vi "delta&2400 measure.vi"(0 "6221":refnum<visa-resource-name>, 5 "2400":refnum<visa-resource-name>, 9 "Timeout":u32, 11 "错误输出":errorcluster) -> (3 "source current":string, 4 "6221":refnum<visa-resource-name>, 6 "2400 resource name out":refnum<visa-resource-name>, 8 "2400":string[](array[string]), 10 "6221":string, 14 "compliance?":bool, 15 "error out":errorcluster)   [LabVIEW 2019, in "nematic.lvlib"]
uses:
  SubVI/nematic.lvlib
  lib/Keithley 622x/Configure/Format/Typedefs/KE622x -- Optional Meas Elements.ctl
  lib/Keithley 622x/Keithley 622x.lvlib
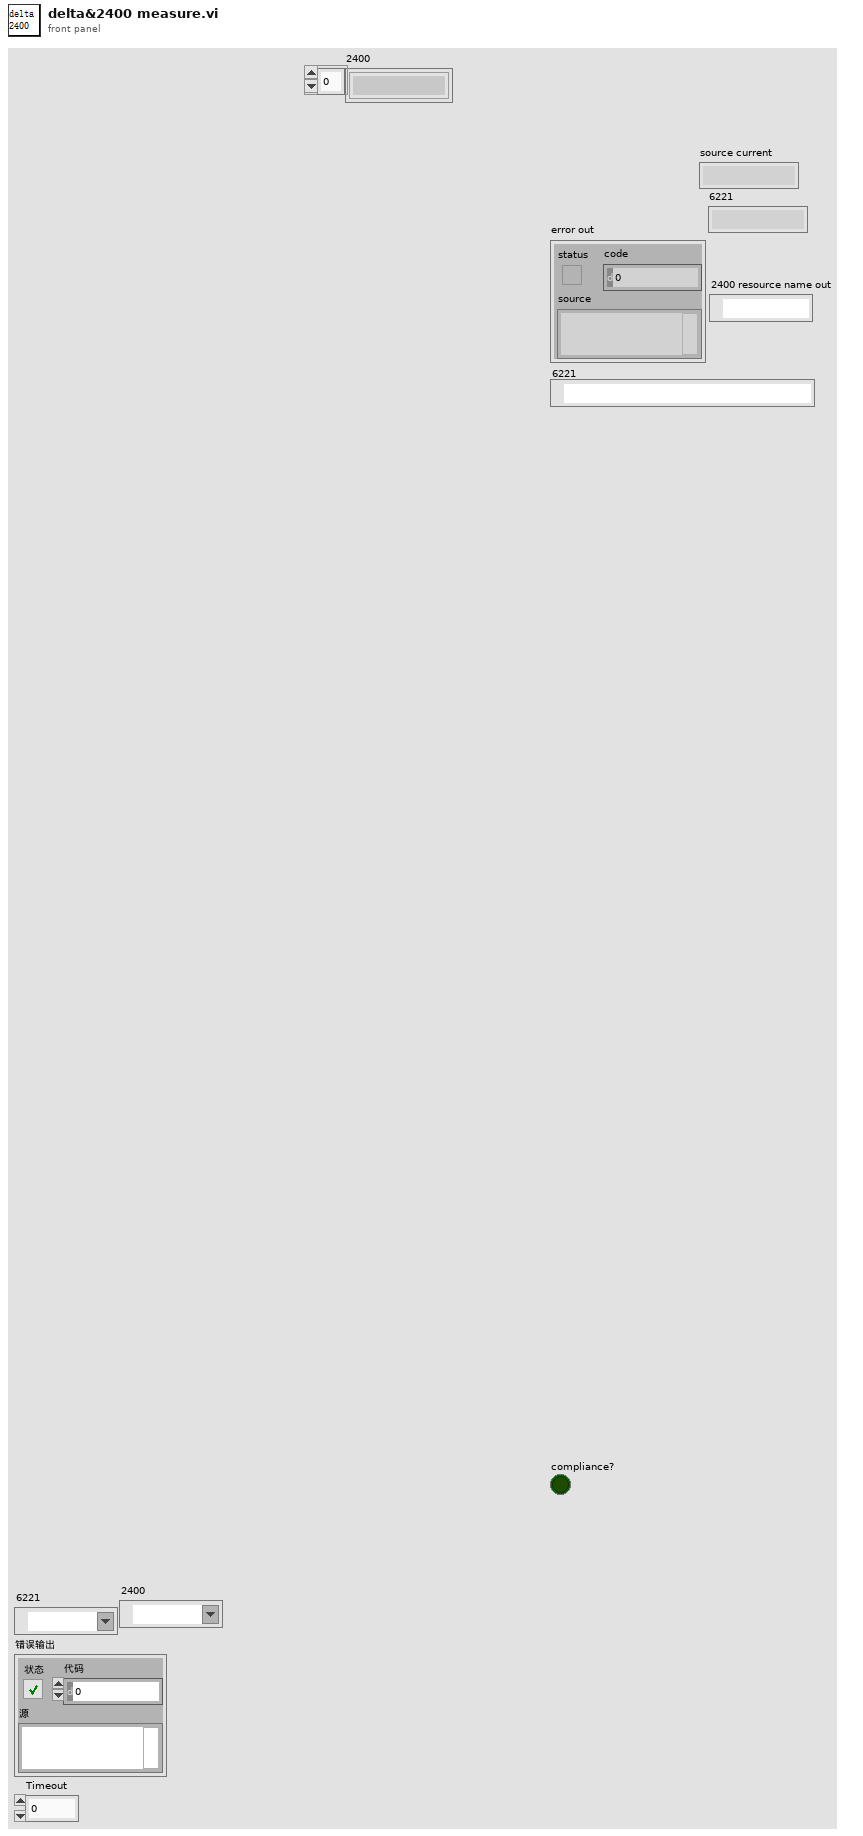
[diagram p1: front panel]
types:
  T1 = typedef "Keithley 622x.lvlib/KE622x -- Optional Meas Elements.ctl" = cluster{"Timstamp?":bool, "Reading Num?":bool, "Source Value?":bool, "Compliance?":bool, "Average Voltage?":bool}
  T2 = typedef "Keithley 622x.lvlib/KE622x -- Meas Event Reg State.ctl" = cluster{"B0, ROF:  KE2182A Delta Reading Overflow Event?":bool, "B1, Int:  Interlock OK Event?":bool, "B2, Temp:  Over Temperature Event?":bool, "B3, Comp:  Compliance Event?":bool, "B5, RAV:  Delta Reading Available Event?":bool, "B6, TN:  User Defined Reading Number Stored In Buffer Event?":bool, "B7, BAV:  At Least 2 Readings Stored In Buffer Event?":bool, "B12, BQF:  Buffer Quarter Full Event?":bool, "B8, BHF:  Buffer Half Full Event?":bool, "B13, B3QF:  Buffer 3/4 Full Event?":bool, "B9, BFL:  Buffer Full Event?":bool}
  T3 = typedef "Keithley 622x.lvlib/KE622x -- Trace Buf.ctl" = cluster{"Additional Valid Arrays":T1, "Reading Num":u32[], "Timestamp (secs)":sgl[], "Source Val (A)":sgl[], "Reading":sgl[], "Average Voltage (V)":sgl[], "Compliance?":bool[]}
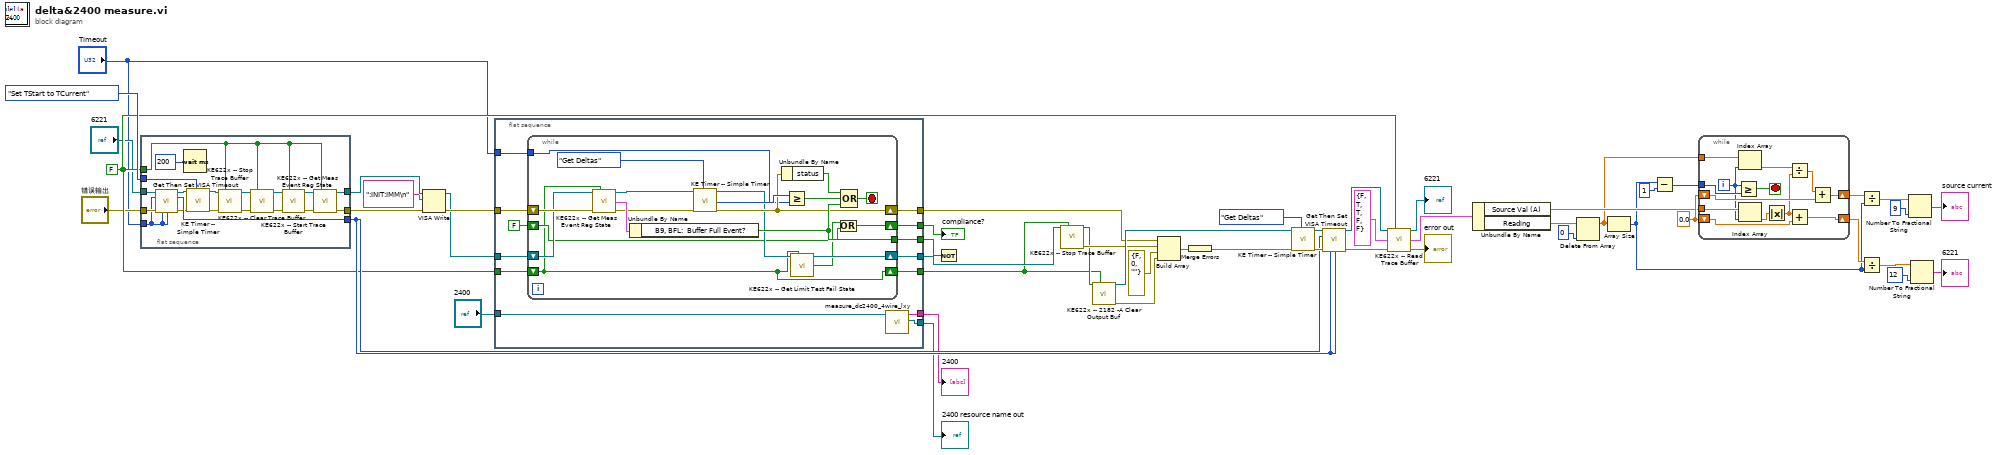
[diagram p0: block diagram]
diagram:
  w20 = FALSE ("Check For SCPI Errors? (T) 2")
  w33 = sgl 0.0 ("Numeric")
  n1 = flat-sequence {
    tunnel: enum16{"Set TStart to TCurrent", "Get Deltas"}."Set TStart to TCurrent" ("Action") -> [w66]
    tunnel: [w53] -> w44
    tunnel: [w52] -> w43
    tunnel: [w61] -> w36
    tunnel: "6221" -> [w58]
    tunnel: w20 -> [w57]
    tunnel: "错误输出" -> [w56]
    tunnel: "Timeout" -> [w55]
    frame #0 {
      n2 = call "Get Then Set VISA Timeout.vi"("VISA Resource Name In"=w58, "New Timeout (msecs)"=w55, "error in (no error)"=w56, "Max Timeout (300 secs)"=w55, "Min Timeout (3 secs)"=w55) -> ("VISA Resource Name Out (dupl)"=w60:refnum<visa-resource-name>, "Old Timeout (msecs)"=w61:u32, "error out"=w59:errorcluster)  [unwired: 7 in, 1 out]
      n3 = Wait (ms)(milliseconds to wait=u32 200) -> ()  [unwired: 1 out]
      n4 = call "KE Timer -- Simple Timer.vi"("Resource In"=w60, "error in (no error)"=w59, "Action"=w66) -> ("Resource Out (dupl)"=w65:refnum<visa-resource-name>, "error out (dupl)"=w64:errorcluster)  [unwired: 7 in, 8 out]
      n5 = call "KE622x -- Stop Trace Buffer.vi"("Resource In"=w65, "Check For SCPI Errors? (T)"=w57, "error in (no error)"=w64) -> ("Resource Out (dupl)"=w70:refnum<visa-resource-name>, "error out"=w69:errorcluster)  [unwired: 11 in]
      n6 = call "KE622x -- Clear Trace Buffer.vi"("Resource In"=w70, "Check For SCPI Errors? (T)"=w57, "error in (no error)"=w69) -> ("Resource Out (dupl)"=w63:refnum<visa-resource-name>, "error out"=w62:errorcluster)  [unwired: 11 in]
      n7 = call "KE622x -- Start Trace Buffer.vi"("Resource In"=w63, "Check For SCPI Errors? (T)"=w57, "error in (no error)"=w62) -> ("Resource Out (dupl)"=w67:refnum<visa-resource-name>, "error out"=w68:errorcluster)  [unwired: 11 in]
      n8 = call "KE622x -- Get Meas Event Reg State.vi"("VISA Resource In"=w67, "Error Query (T)?"=w57, "error in (no error)"=w68) -> ("VISA Resource Out (dupl)"=w53:refnum<visa-resource-name>, "error out"=w52:errorcluster)  [unwired: 10 in, 1 out]
    }
  }
  n9 = VISA Write(VISA resource name=w44, write buffer=":INIT:IMM\n", error in (no error)=w43) -> (VISA resource name out=w21:refnum<visa-resource-name>, error out=w22:errorcluster)  [unwired: 1 out]
  n10 = flat-sequence {
    tunnel: [w71] -> w8
    tunnel: [w72] -> w9
    tunnel: "2400" -> [w73]
    tunnel: "Timeout" -> [w75]
    tunnel: [w76] -> w10
    tunnel: [w77] -> w16
    tunnel: [w78] -> w17
    tunnel: [w79] -> w18
    tunnel: [w80] -> w19
    tunnel: w20 -> [w81]
    tunnel: w21 -> [w82]
    tunnel: w22 -> [w83]
    frame #0 {
      n11 = while {
        shift-right: [w93] -> w80
        shift-left: w83 -> [w102]
        shift-right: [w89] -> w79
        shift-left: w82 -> [w101]
        tunnel: [w95] -> w78
        shift-right: [w85] -> w77
        shift-left: w81 -> [w85]
        tunnel: w75 -> [w91]
        shift-right: [w87] -> w76
        shift-left: FALSE -> [w86]
        stop <- w84 stop-if-true
        n12 = call "KE622x -- Get Meas Event Reg State.vi"("VISA Resource In"=w101, "Error Query (T)?"=w85, "error in (no error)"=w102) -> ("VISA Resource Out (dupl)"=w98:refnum<visa-resource-name>, "KE622x Meas Event Reg"=w100:T2, "error out"=w99:errorcluster)  [unwired: 10 in]
        n13 = Unbundle By Name(w100) -> ("B9, BFL:  Buffer Full Event?"=w95:bool)
        n14 = call "KE Timer -- Simple Timer.vi"("Resource In"=w98, "error in (no error)"=w99, "Action"=enum16{"Set TStart to TCurrent", "Get Deltas"}."Get Deltas") -> ("Resource Out (dupl)"=w90:refnum<visa-resource-name>, "TCurrent - TStart (ms)"=w96:u32, "error out (dupl)"=w93:errorcluster)  [unwired: 7 in, 7 out]
        n15 = Unbundle By Name(w93) -> ("status"=w92:bool)
        n16 = Greater Or Equal?(x=w96, y=w91) -> (x >= y?=w94:bool)
        n17 = call "KE622x -- Get Limit Test Fail State.vi"("Resource In"=w90, "Check For SCPI Errors? (T)"=w85) -> ("Resource Out (dupl)"=w89:refnum<visa-resource-name>, "Limit Test Failed (Compliance)?"=w88:bool)  [unwired: 11 in, 1 out]
        n18 = Or(x=w88, y=w86) -> (x .or. y?=w87:bool)
        n19 = Compound Arithmetic op=OR(w92, w94, w95) -> (w84:bool)
      }
      n20 = call "measure_dc2400_4wire_lxy.vi"("2400 resource name"=w73) -> ("2400 resource name out"=w71:refnum<visa-resource-name>, "输出数组"=w72:string[])  [unwired: 8 in, 1 out]
    }
  }
  n21 = Not(x=w17) -> ()  [unwired: 1 out]
  n22 = call "KE622x -- Stop Trace Buffer.vi"("Resource In"=w18, "Check For SCPI Errors? (T)"=w16) -> ("Resource Out (dupl)"=w28:refnum<visa-resource-name>, "error out"=w41:errorcluster)  [unwired: 12 in]
  n23 = call "KE622x -- 2182 -A Clear Output Buf.vi"("622x Resource In"=w28, "Check For SCPI Errors? (T)"=w16) -> ("622x Resource Out (dupl)"=w46:refnum<visa-resource-name>, "error out"=w40:errorcluster)  [unwired: 11 in, 1 out]
  n24 = Build Array(w19, w41, errorcluster {"status"=FALSE, "code"=0, "source"=""} ("error out"), w40) -> (w42:errorcluster[])
  n25 = Merge Errors(w42) -> (w39:errorcluster)
  n26 = call "KE Timer -- Simple Timer.vi"("Resource In"=w46, "error in (no error)"=w39, "Action"=enum16{"Set TStart to TCurrent", "Get Deltas"}."Get Deltas") -> ("Resource Out (dupl)"=w37:refnum<visa-resource-name>, "error out (dupl)"=w38:errorcluster)  [unwired: 7 in, 8 out]
  n27 = call "Get Then Set VISA Timeout.vi"("VISA Resource Name In"=w37, "New Timeout (msecs)"=w36, "error in (no error)"=w38, "Max Timeout (300 secs)"=w36, "Min Timeout (3 secs)"=w36) -> ("VISA Resource Name Out (dupl)"=w35:refnum<visa-resource-name>, "error out"=w34:errorcluster)  [unwired: 7 in, 2 out]
  n28 = call "KE622x -- Read Trace Buffer.vi"("Resource In"=w35, "Check For SCPI Errors? (T)"=w20, "Meas Elements To Return"=T1 {"Timstamp?"=FALSE, "Reading Num?"=TRUE, "Source Value?"=TRUE, "Compliance?"=FALSE, "Average Voltage?"=FALSE}, "error in (no error)"=w34) -> ("Resource Out (dupl)"=→"6221":refnum<visa-resource-name>, "Trace Buf"=w51:T3, "error out"=→"error out":errorcluster)  [unwired: 9 in]
  n29 = Unbundle By Name(w51) -> ("Source Val (A)"=w31:sgl[], "Reading"=w24:sgl[])
  n30 = Delete From Array(array=w24, index=0 ("索引")) -> (array with subset deleted=w23:sgl[])  [unwired: 1 in, 1 out]
  n31 = Array Size(array=w23) -> (size(s)=w30:i32)
  n32 = Subtract(x=w30, y=1) -> (x-y=w48:i32)
  n33 = while {
    tunnel: w23 -> [w115]
    shift-right: [w113] -> w50
    shift-left: w33 -> [w114]
    tunnel: w48 -> [w112]
    tunnel: w31 -> [w110]
    shift-right: [w107] -> w32
    shift-left: w33 -> [w108]
    i -> [w109]
    stop <- w111 stop-if-true
    n34 = Greater Or Equal?(x=w109, y=w112) -> (x >= y?=w111:bool)
    n35 = Index Array(array=w115, index=w109) -> (element=w106:sgl)
    n36 = Index Array(array=w110, index=w109) -> (element=w105:sgl)
    n37 = Absolute Value(x=w105) -> (abs(x)=w103:sgl)
    n38 = Divide(x=w106, y=w103) -> (x/y=w104:sgl)
    n39 = Add(x=w103, y=w108) -> (x+y=w107:sgl)
    n40 = Add(x=w104, y=w114) -> (x+y=w113:sgl)
  }
  n41 = Divide(x=w50, y=w30) -> (x/y=w5:sgl)
  n42 = Divide(x=w32, y=w30) -> (x/y=w2:sgl)
  n43 = Number To Fractional String(number=w5, precision (6)=i16 9 ("精度(6)")) -> (F-format string=→"source current":string)  [unwired: 2 in]
  n44 = Number To Fractional String(number=w2, precision (6)=i16 12) -> (F-format string=→"6221":string)  [unwired: 2 in]
  "2400 resource name out" <- w8
  "compliance?" <- w10
  "2400" <- w9
